vi "laser power FGV.vi"(6 "Mode":T1(ring), 9 "laser index":u16, 11 "Input power":dbl) -> (3 "Output power":dbl)   [LabVIEW 2018, in "Application.lvlib"]
uses:
  Application.lvlib
panel:
  out "Array":dbl[](array[numeric])
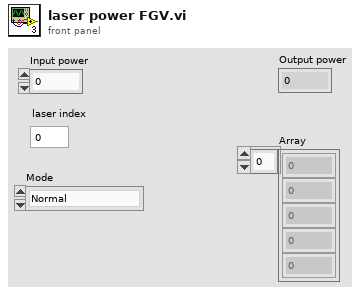
[diagram p1: front panel]
types:
  T1 = enum16{"Normal", "Ignore", "Reset", "Initialize"}
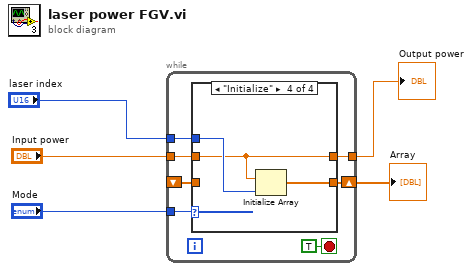
[diagram p0: block diagram]
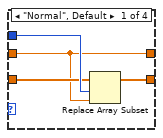
[diagram p2: hidden frame]
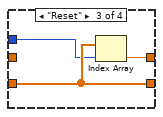
[diagram p4: hidden frame]
diagram:
  n1 = while {
    shift-right: [w10] -> w5
    shift-left: _ -> [w11]
    tunnel: "Mode" -> [w9]
    tunnel: "Input power" -> [w8]
    tunnel: [w7] -> w1
    tunnel: "laser index" -> [w6]
    stop <- TRUE stop-if-true
    n2 = case shown="\"Initialize\"" w9 {
      tunnel: w11 -> [w15 w18 w21 _]
      tunnel: [w14 w18 w21 w23] -> w10
      tunnel: w8 -> [w13 w17 _ w22]
      tunnel: [w13 w17 w19 w22] -> w7
      tunnel: w6 -> [w16 _ w20 w24]
      frame "Normal", Default {
        n3 = Replace Array Subset(array=w15, new element=w13, index=w16) -> (w14:dbl[])
      }
      frame "Ignore" {
      }
      frame "Reset" {
        n4 = Index Array(array=w21, index=w20) -> (element=w19:dbl)
      }
      frame "Initialize" {
        n5 = Initialize Array(w22, w24) -> (w23:dbl[])
      }
    }
  }
  "Array" <- w5
  "Output power" <- w1
